vi "SVL Max-Min Level (resampled) (N Ch).vi"(6 "restart averaging (F)":bool, 8 "error in (no error)":errorcluster, 10 "even-angle channel info":T1[](array[typedef]) {"channel info"."pregain" format="%.2f"; "channel info"."weighting filter" items=["Linear", "A-weighting", "B-weighting", "C-weighting", "ITU-R 468-4", "Dolby", "CCITT", "C-message", "Wb", "Wc", "Wd", "We", "Wf", "Wh", "Wj", "Wk", "Wm", "AES17 20 kHz lowpass", "AES17 40 kHz lowpass", "AES17 20 kHz highpass", "AES17 40 kHz highpass"]; "channel info"."dB reference" format="%^.1e"; "channel info"."engineering units" items=["custom..."=0, "V"=1, "A"=21, "C"=30, "pC"=31, "s"=32, "-"=29, "Pa"=2, "N"=20, "g"=3, "m/s^2"=4, "m/s"=5, "m"=6, "mm/s"=12, "mm"=13, "micron/s"=14, "micron"=15, "in/s^2"=7, "in/s"=8, "in"=9, "mil/s"=10, "mil"=11, "rad/s^2"=16, "rad/s"=17, "rad"=18, "deg/s^2"=26, "deg/s"=27, "deg"=28, "RPM"=22, "cycle/s^2"=23, "Hz"=24, "cycle"=25, "strain"=19]; "channel info"."sensor sensitivity" format="%#_5f"}, 11 "even-angle signals [EU]":T5(array[cluster]) {"even-angle signal" format="%.2f"; "dr" format="%.2f"; "r0" format="%.2f"}) -> (0 "error out":errorcluster, 2 "unit labels":string[](array[string]), 3 "max-min levels [EU]":dbl[](array[numeric]) format="%.2f", 5 "min levels [EU]":dbl[](array[numeric]) format="%.2f", 7 "max levels [EU]":dbl[](array[numeric]) format="%.2f")   [LabVIEW 2017, in "SoundVib_VibrationLevel.lvlib"]
doc: "Computes the maximum and minimum levels of all previous values and the difference between the maximum and minimum levels of <B>scaled signal [EU]</B> or <B>even-angle signal [EU]</B>. <B>scaled signal [EU]</B> should have a zero DC component. You can attenuate the DC component with hardware AC-coupling filters and with software high-pass filters. Wire data to the <B>scaled signal [EU]</B> input to determine the polymorphic instance to use or manually select the instance."
uses:
  <vilib>/addons/Sound and Vibration/svt_Level/SoundVib_VibrationLevel.lvlib
  <vilib>/addons/_NISVFA/_Shared subVIs/Controls/svc_Resampled Channel Info.ctl
  <vilib>/addons/_NISVFA/_Shared subVIs/Controls/svc_Channel Info.ctl
  <vilib>/addons/_NISVFA/_Shared subVIs/Controls/svc_Engineering Units Text Ring.ctl
  <vilib>/addons/_NISVFA/_Shared subVIs/Controls/svc_Weighting Filter Text Ring.ctl
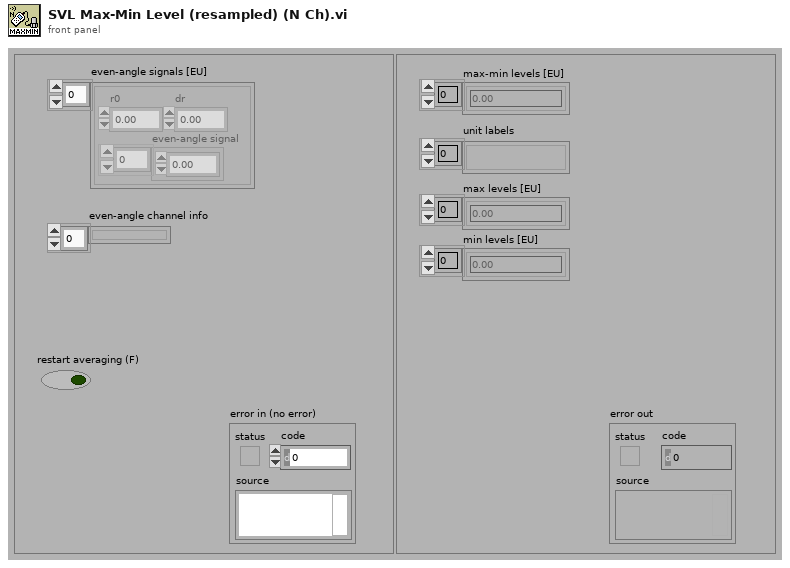
[diagram p1: front panel]
types:
  T1 = typedef "svc_Resampled Channel Info.ctl" = cluster{"channel name":string, "description":string, " channel info":T2}
  T2 = typedef "svc_Channel Info.ctl" = cluster{"sensor sensitivity":dbl, "engineering units":T3, "dB reference":dbl, "custom label":string, "weighting filter":T4, "pregain":dbl}
  T3 = typedef "svc_Engineering Units Text Ring.ctl" = u16
  T4 = typedef "svc_Weighting Filter Text Ring.ctl" = u16
  T5 = cluster{"r0":dbl, "dr":dbl, "even-angle signal":dbl[]}[]
  T6 = enum16{"RMS", "Running RMS", "Exp avg  ", "Dec exp avg ", "Peak", "Crest"}
  T7 = cluster{"r0":dbl, "dr":dbl, "even angle signal":dbl[]}[]
  T8 = enum16{"Reset filter", "Restart averaging", "Continue processing"}
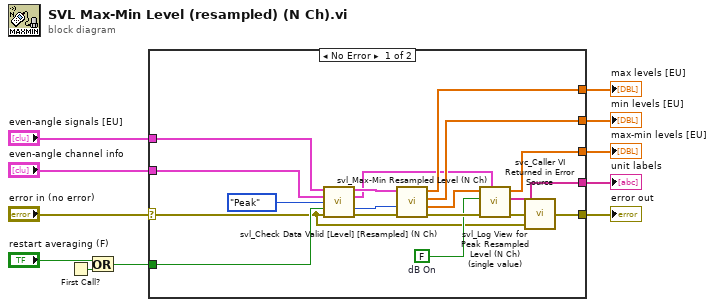
[diagram p0: block diagram]
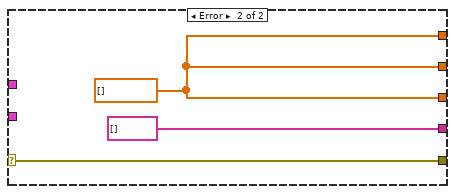
[diagram p2: hidden frame]
diagram:
  n1 = First Call?() -> (First Call?: T/F=w7:bool)
  n2 = Or(x="restart averaging (F)", y=w7) -> (x .or. y?=w5:bool)
  n3 = case shown="No Error" "error in (no error)" {
    selector: "error in (no error)" -> [w12 w32]
    tunnel: [w25 w32] -> w11
    tunnel: [w28 string[] [] ("unit label [ ]")] -> w10
    tunnel: [w27 w30] -> w9
    tunnel: "even-angle signals [EU]" -> [w14 _]
    tunnel: w5 -> [w23 _]
    tunnel: [w21 w30] -> w3
    tunnel: [w20 w30] -> w2
    tunnel: "even-angle channel info" -> [w15 _]
    frame No Error {
      w17 = FALSE  # dB On
      n4 = call <vilib>:"svl_Check Data Valid [Level] [Resampled] (N Ch).vi"("scaled even angle signals [EU]"=w14, "even angle channel info"=w15, "level analysis"=T6."Peak" ("Level Analysis"), "restart averaging (F)"=w23, "error in (no error)"=w12) -> ("dup scaled even angle signals [EU]"=w16:T7, "dup even angle channel info"=w13:T1[], "processing state"=w22:T8, "error out"=w24:errorcluster)  [unwired: 7 in]
      n5 = call <vilib>:"svl_Max-Min Resampled Level (N Ch).vi"("error in (no error)"=w24, "processing state"=w22, "even angle signals"=w16) -> ("error out"=w26:errorcluster, "max-min level(s)"=w18:dbl[], "min level(s)"=w20:dbl[], "max level(s)"=w21:dbl[])  [unwired: 5 in]
      n6 = call <vilib>:"svl_Log View for Peak Resampled Level (N Ch) (single value).vi"("even angle channel info"=w13, "error in (no error)"=w26, "dB On (T)"=w17, "peak levels [EU]"=w18) -> ("error out"=w29:errorcluster, "unit label [ ]"=w28:string[], "peak levels [EU]"=w27:dbl[])  [unwired: 5 in]
      n7 = call <vilib>:"svc_Caller VI Returned in Error Source.vi"("warning input to caller"=w12, "error in (no error)"=w29) -> ("error out"=w25:errorcluster)  [unwired: 3 in]
    }
    frame Error {
      w30 = dbl[] [] ("energy levels [EU^2 rms]")
    }
  }
  "max-min levels [EU]" <- w9
  "unit labels" <- w10
  "error out" <- w11
  "max levels [EU]" <- w3
  "min levels [EU]" <- w2
